vi "UART Close.vi"(8 "Error In":errorcluster, 10 "UART Channel":u8, 11 "LINX Device Config":T1) -> (0 "Error Out":errorcluster, 3 "LINX Device Config":T1)   [LabVIEW 2014, in "LMH-LINX.lvlib" / "Device.lvlib"]
doc: "Close the specified UART channel."
uses:
  <vilib>/MakerHub/LINX/Private/Device/Device.lvlib
  <vilib>/MakerHub/LINX/Private/Device/Type Defs/LINX Device Config.ctl
  <vilib>/MakerHub/LINX/Private/Type Defs/Interface.ctl
  <vilib>/MakerHub/LINX/Private/Device/Type Defs/TCP Config.ctl
  <vilib>/MakerHub/LINX/Private/Device/Type Defs/Channels.ctl
  <vilib>/MakerHub/LINX/Private/Type Defs/Error Type.ctl
  <vilib>/MakerHub/LINX/LMH-LINX.lvlib
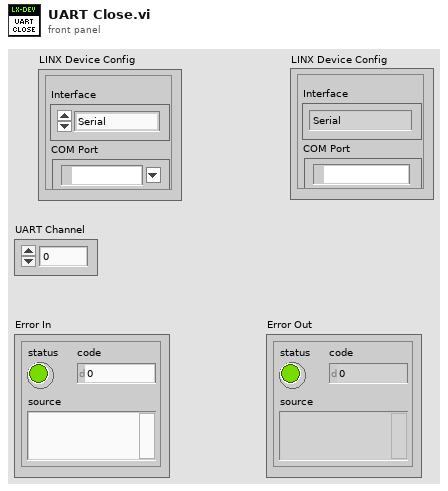
[diagram p1: front panel]
types:
  T1 = typedef "LMH-LINX.lvlib/Device.lvlib/LINX Device Config.ctl" = cluster{"Interface":T2, "COM Port":refnum<visa-resource-name>, "TCP Configuration":T3, "Device Family":u8, "Device ID":u8, "Device Name":string, "TCP Ref":refnum<k5>, "Channels":T4}
  T2 = typedef "LMH-LINX.lvlib/Interface.ctl" = enum16{"Serial", "TCP"}
  T3 = typedef "LMH-LINX.lvlib/Device.lvlib/TCP Config.ctl" = cluster{"IP Address":string, "Port":u16}
  T4 = typedef "LMH-LINX.lvlib/Channels.ctl" = cluster{"DI":u8[], "DO":u8[], "AI":u8[], "AO":u8[], "PWM":u8[], "QE":u8[], "UART":u8[], "I2C 2":u8[], "SPI":u8[], "CAN":u8[], "Servo":u8[], "AI Ref (V)":dbl, "AI Resolution (Bits)":u8, "AO Ref (V)":dbl, "AO Resolution (Bits)":u8}
  T5 = typedef "LMH-LINX.lvlib/Error Type.ctl" = enum16{"Unknown", "Timeout", "Corrupt Return Packet", "Unable To Connect", "Command Not Supported", "Channel DNE", "Invalid COM Config", "Firmware Version Mismatch", "myRIO Support", "CMD Specific Error", "Local IO Not Supported"}
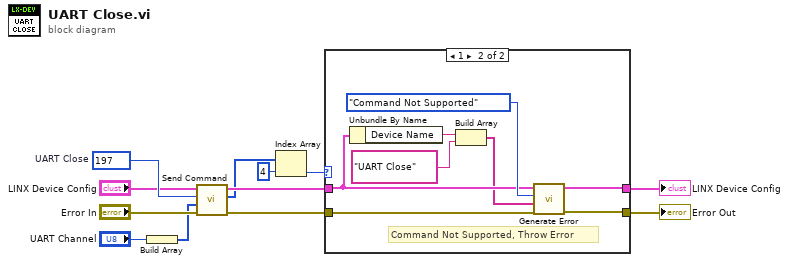
[diagram p0: block diagram]
diagram:
  w11 = u16 197  # UART Close
  n1 = Build Array("UART Channel") -> (w2:u8[])
  n2 = call <vilib>:"Send Command.vi"("Error In"="Error In", "ARGS"=w2, "CMD"=w11, "LINX Device Config"="LINX Device Config") -> ("Error Out"=w4:errorcluster, "Response"=w1:u8[], "LINX Device Config"=w6:T1)  [unwired: 4 in, 1 out]
  n3 = Index Array(array=w1, index=4) -> (element=w8:u8)
  n4 = case shown="1" w8 {
    tunnel: [w14 w20] -> w7
    tunnel: w6 -> [w14 w16]
    tunnel: [w13 w21] -> w5
    tunnel: w4 -> [w13 w22]
    frame 0, Default {
      # "Status OK, Process Data"
    }
    frame 1 {
      # "Command Not Supported, Throw Error"
      n5 = Unbundle By Name(w16) -> ("Device Name"=w18:string)
      n6 = Build Array(w18, "UART Close") -> (w15:string[])
      n7 = call <vilib>:"Generate Error.vi"("Error In"=w22, "Arguments"=w15, "Error Type"=Error_Type."Command Not Supported", "LINX Device Config"=w16) -> ("Error Out"=w21:errorcluster, "Dup LINX Device Config"=w20:T1)  [unwired: 6 in]
    }
  }
  "Error Out" <- w5
  "LINX Device Config" <- w7
